vi "Configure Alternation Trigger (Glitch).vi"(0 "VISA resource name":refnum<visa-resource-name>, 1 "Glitch Polarity (0: Positive)":u16(ring) items=["Positive", "Negative"], 5 "Trigger Source (0: Source A)":u16(ring) items=["Source A", "Source B"], 7 "Glitch Condition (0: Less Than)":u16(ring) items=["Less Than", "Greater Than"], 9 "Glitch Width (1E-5 s)":dbl=1e-05, 11 "error in (no error)":errorcluster) -> (4 "VISA resource name out":refnum<visa-resource-name>, 15 "error out":errorcluster)   [LabVIEW 2010, in "Agilent DSO1000 Series.lvlib"]
doc: "Configures the glitch trigger under alternation trigger mode. A glitch trigger occurs when the trigger signal has a pulse with a width that is less than,greater than or equal to the glitch width based on the \"Glitch Mode\" control. You specify the glitch width in the \"Glitch Width\" control. You specify the polarity of the pulse with the \"Glitch Polarity\" control."
uses:
  <instrlib>/Agilent DSO1000 Series/Agilent DSO1000 Series.lvlib
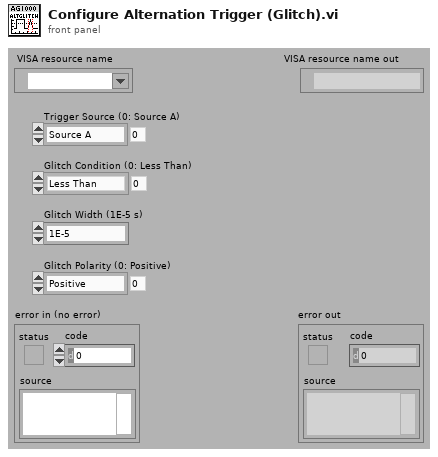
[diagram p1: front panel]
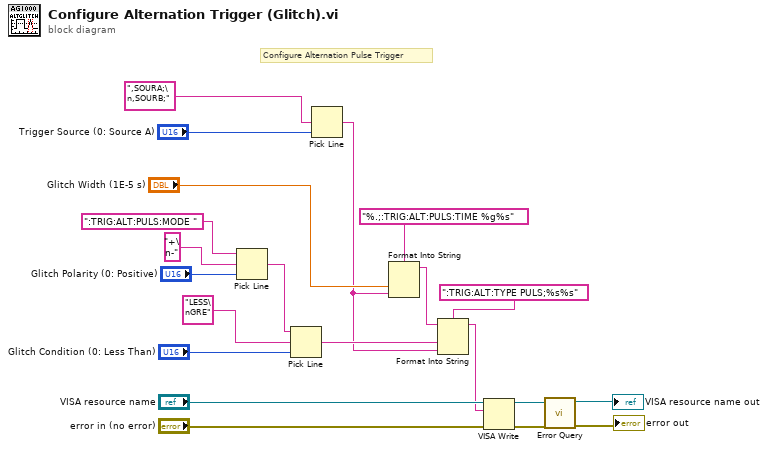
[diagram p0: block diagram]
diagram:
  # "Configure Alternation Pulse Trigger"
  n1 = Pick Line(string ("")=":TRIG:ALT:PULS:MODE ", multi-line string="+\n-", line index="Glitch Polarity (0: Positive)") -> (output string=w15:string)
  n2 = Pick Line(string ("")=w15, multi-line string="LESS\nGRE", line index="Glitch Condition (0: Less Than)") -> (output string=w3:string)
  n3 = Pick Line(multi-line string=",SOURA;\n,SOURB;", line index="Trigger Source (0: Source A)") -> (output string=w2:string)  [unwired: 1 in]
  n4 = Format Into String(format string="%.;:TRIG:ALT:PULS:TIME %g%s", "Glitch Width (1E-5 s)", w2) -> (resulting string=w4:string)  [unwired: 2 in, 1 out]
  n5 = Format Into String(format string=":TRIG:ALT:TYPE PULS;%s%s", initial string=w4, w3, w2) -> (resulting string=w1:string)  [unwired: 1 in, 1 out]
  n6 = VISA Write(VISA resource name="VISA resource name", write buffer=w1, error in (no error)="error in (no error)") -> (VISA resource name out=w10:refnum<visa-resource-name>, error out=w11:errorcluster)  [unwired: 1 out]
  n7 = call <instrlib>:"Error Query.vi"("error in (no error)"=w11, "VISA resource name"=w10) -> ("error out"=→"error out":errorcluster, "VISA resource name out"=→"VISA resource name out":refnum<visa-resource-name>)  [unwired: 6 in, 2 out]
